vi "Start.vi"() -> ()   [LabVIEW 2016]
panel:
  in  "initial instruction string":string
  out "return count":u32=6435
  out "appended instruction string 2":string="dds reset\rdcp spi:CFR1=0x404000\rdcp spi:CFR2=0x80080\rdcp 0 spi:STP0=0x3FFF0000028F5C29\rdcp 1 spi:STP0=0x3FFF0000028F5C29\rdcp 0 spi:DRL=0x147C0118147BC1DB\rdcp 0 spi:DRSS=0xFFFFFFFF00000003\rdcp 0 spi:DRR=0x2D3E\rdcp 0 update:u-d\rdcp 0 update:+d\rdcp 1 spi:DRL=0x147AE148147AE148\rdcp 1 spi:DRSS=0xFFFFFFFF00000000\rdcp 1 spi:DRR=0xFFFF\rdcp 1 update:u-d\rdcp 1 update:+d\rdcp wait:1h:\rdcp wait::DROVER\rdcp 0 spi:DRL=0x147C51F1147C0118\rdcp 0 spi:DRSS=0xFFFFFFFF00000004\rdcp 0 spi:DRR=0x2F2F\rdcp 0 update:u-d\rdcp 0 update:+d\rdcp wait:1h:\rdcp wait::DROVER\rdcp 0 spi:DRL=0x147CB92D147C51F1\rdcp 0 spi:DRSS=0xFFFFFFFF00000017\rdcp 0 spi:DRR=0xD478\rdcp 0 update:u-d\rdcp 0 update:+d\rdcp wait:1h:\rdcp wait::DROVER\rdcp 0 spi:DRL=0x147D3CCC147CB92D\rdcp 0 spi:DRSS=0xFFFFFFFF00000009\rdcp 0 spi:DRR=0x4136\rdcp 0 update:u-d\rdcp 0 update:+d\rdcp wait:1h:\rdcp wait::DROVER\rdcp 0 spi:DRL=0x147DE446147D3CCC\rdcp 0 spi:DRSS=0xFFFFFFFF0000000D\rdcp 0 spi:DRR=0x4A07\rdcp 0 update:u-d\rdcp 0 update:+d\rdcp wait:1h:\rdcp wait::DROVER\rdcp 0 spi:DRL=0x147EB8D6147DE446\rdcp 0 spi:DRSS=0xFFFFFFFF0000002B\rdcp 0 spi:DRR=0xC0EC\rdcp 0 update:u-d\rdcp 0 update:+d\rdcp wait:1h:\rdcp wait::DROVER\rdcp 0 spi:DRL=0x147FC5C3147EB8D6\rdcp 0 spi:DRSS=0xFFFFFFFF00000006\rdcp 0 spi:DRR=0x1547\rdcp 0 update:u-d\rdcp 0 update:+d\rdcp wait:1h:\rdcp wait::DROVER\rdcp 0 spi:DRL=0x148118A1147FC5C3\rdcp 0 spi:DRSS=0xFFFFFFFF0000001C\rdcp 0 spi:DRR=0x4ECD\rdcp 0 update:u-d\rdcp 0 update:+d\rdcp wait:1h:\rdcp wait::DROVER\rdcp 0 spi:DRL=0x1482C174148118A1\rdcp 0 spi:DRSS=0xFFFFFFFF00000049\rdcp 0 spi:DRR=0xA3E0\rdcp 0 update:u-d\rdcp 0 update:+d\rdcp wait:1h:\rdcp wait::DROVER\rdcp 0 spi:DRL=0x1484D2A81482C174\rdcp 0 spi:DRSS=0xFFFFFFFF00000003\rdcp 0 spi:DRR=0x568\rdcp 0 update:u-d\rdcp 0 update:+d\rdcp wait:1h:\rdcp wait::DROVER\rdcp 0 spi:DRL=0x148760AD1484D2A8\rdcp 0 spi:DRSS=0xFFFFFFFF0000008C\rdcp 0 spi:DRR=0xCC25\rdcp 0 update:u-d\rdcp 0 update:+d\rdcp wait:1h:\rdcp wait::DROVER\rdcp 0 spi:DRL=0x148A8111148760AD\rdcp 0 spi:DRSS=0xFFFFFFFF00000049\rdcp 0 spi:DRR=0x56FB\rdcp 0 update:u-d\rdcp 0 update:+d\rdcp wait:1h:\rdcp wait::DROVER\rdcp 0 spi:DRL=0x148E48EB148A8111\rdcp 0 spi:DRSS=0xFFFFFFFF00000004\rdcp 0 spi:DRR=0x3F1\rdcp 0 update:u-d\rdcp 0 update:+d\rdcp wait:1h:\rdcp wait::DROVER\rdcp 0 spi:DRL=0x1492CA77148E48EB\rdcp 0 spi:DRSS=0xFFFFFFFF000000A0\rdcp 0 spi:DRR=0x8447\rdcp 0 update:u-d\rdcp 0 update:+d\rdcp wait:1h:\rdcp wait::DROVER\rdcp 0 spi:DRL=0x149811DB1492CA77\rdcp 0 spi:DRSS=0xFFFFFFFF000000D0\rdcp 0 spi:DRR=0x92C9\rdcp 0 update:u-d\rdcp 0 update:+d\rdcp wait:1h:\rdcp wait::DROVER\rdcp 0 spi:DRL=0x149E2175149811DB\rdcp 0 spi:DRSS=0xFFFFFFFF00000100\rdcp 0 spi:DRR=0x9D59\rdcp 0 update:u-d\rdcp 0 update:+d\rdcp wait:1h:\rdcp wait::DROVER\rdcp 0 spi:DRL=0x14A4EE42149E2175\rdcp 0 spi:DRSS=0xFFFFFFFF000000C7\rdcp 0 spi:DRR=0x6D05\rdcp 0 update:u-d\rdcp 0 update:+d\rdcp wait:1h:\rdcp wait::DROVER\rdcp 0 spi:DRL=0x14AC5D7114A4EE42\rdcp 0 spi:DRSS=0xFFFFFFFF00000019\rdcp 0 spi:DRR=0xC87\rdcp 0 update:u-d\rdcp 0 update:+d\rdcp wait:1h:\rdcp wait::DROVER\rdcp 0 spi:DRL=0x14B4443314AC5D71\rdcp 0 spi:DRSS=0xFFFFFFFF00000021\rdcp 0 spi:DRR=0xF8F\rdcp 0 update:u-d\rdcp 0 update:+d\rdcp wait:1h:\rdcp wait::DROVER\rdcp 0 spi:DRL=0x14BC6A7F14B44433\rdcp 0 spi:DRSS=0xFFFFFFFF0000014D\rdcp 0 spi:DRR=0x9838\rdcp 0 update:u-d\rdcp 0 update:+d\rdcp wait:1h:\rdcp wait::DROVER\rdcp 0 spi:DRL=0x14C490CB14BC6A7F\rdcp 0 spi:DRSS=0xFFFFFFFF0000014D\rdcp 0 spi:DRR=0x9838\rdcp 0 update:u-d\rdcp 0 update:+d\rdcp wait:1h:\rdcp wait::DROVER\rdcp 0 spi:DRL=0x14CC778D14C490CB\rdcp 0 spi:DRSS=0xFFFFFFFF00000021\rdcp 0 spi:DRR=0xF8F\rdcp 0 update:u-d\rdcp 0 update:+d\rdcp wait:1h:\rdcp wait::DROVER\rdcp 0 spi:DRL=0x14D3E6BC14CC778D\rdcp 0 spi:DRSS=0xFFFFFFFF00000019\rdcp 0 spi:DRR=0xC87\rdcp 0 update:u-d\rdcp 0 update:+d\rdcp wait:1h:\rdcp wait::DROVER\rdcp 0 spi:DRL=0x14DAB38914D3E6BC\rdcp 0 spi:DRSS=0xFFFFFFFF000000C7\rdcp 0 spi:DRR=0x6D05\rdcp 0 update:u-d\rdcp 0 update:+d\rdcp wait:1h:\rdcp wait::DROVER\rdcp 0 spi:DRL=0x14E0C32314DAB389\rdcp 0 spi:DRSS=0xFFFFFFFF00000100\rdcp 0 spi:DRR=0x9D59\rdcp 0 update:u-d\rdcp 0 update:+d\rdcp wait:1h:\rdcp wait::DROVER\rdcp 0 spi:DRL=0x14E60A8714E0C323\rdcp 0 spi:DRSS=0xFFFFFFFF000000D0\rdcp 0 spi:DRR=0x92C9\rdcp 0 update:u-d\rdcp 0 update:+d\rdcp wait:1h:\rdcp wait::DROVER\rdcp 0 spi:DRL=0x14EA8C1314E60A87\rdcp 0 spi:DRSS=0xFFFFFFFF000000A0\rdcp 0 spi:DRR=0x8447\rdcp 0 update:u-d\rdcp 0 update:+d\rdcp wait:1h:\rdcp wait::DROVER\rdcp 0 spi:DRL=0x14EE53ED14EA8C13\rdcp 0 spi:DRSS=0xFFFFFFFF00000004\rdcp 0 spi:DRR=0x3F1\rdcp 0 update:u-d\rdcp 0 update:+d\rdcp wait:1h:\rdcp wait::DROVER\rdcp 0 spi:DRL=0x14F1745114EE53ED\rdcp 0 spi:DRSS=0xFFFFFFFF00000049\rdcp 0 spi:DRR=0x56FB\rdcp 0 update:u-d\rdcp 0 update:+d\rdcp wait:1h:\rdcp wait::DROVER\rdcp 0 spi:DRL=0x14F4025514F17451\rdcp 0 spi:DRSS=0xFFFFFFFF0000008C\rdcp 0 spi:DRR=0xCC25\rdcp 0 update:u-d\rdcp 0 update:+d\rdcp wait:1h:\rdcp wait::DROVER\rdcp 0 spi:DRL=0x14F6138A14F40255\rdcp 0 spi:DRSS=0xFFFFFFFF00000003\rdcp 0 spi:DRR=0x568\rdcp 0 update:u-d\rdcp 0 update:+d\rdcp wait:1h:\rdcp wait::DROVER\rdcp 0 spi:DRL=0x14F7BC5D14F6138A\rdcp 0 spi:DRSS=0xFFFFFFFF00000049\rdcp 0 spi:DRR=0xA3E0\rdcp 0 update:u-d\rdcp 0 update:+d\rdcp wait:1h:\rdcp wait::DROVER\rdcp 0 spi:DRL=0x14F90F3B14F7BC5D\rdcp 0 spi:DRSS=0xFFFFFFFF0000001C\rdcp 0 spi:DRR=0x4ECD\rdcp 0 update:u-d\rdcp 0 update:+d\rdcp wait:1h:\rdcp wait::DROVER\rdcp 0 spi:DRL=0x14FA1C2814F90F3B\rdcp 0 spi:DRSS=0xFFFFFFFF00000006\rdcp 0 spi:DRR=0x1547\rdcp 0 update:u-d\rdcp 0 update:+d\rdcp wait:1h:\rdcp wait::DROVER\rdcp 0 spi:DRL=0x14FAF0B814FA1C28\rdcp 0 spi:DRSS=0xFFFFFFFF0000002B\rdcp 0 spi:DRR=0xC0EC\rdcp 0 update:u-d\rdcp 0 update:+d\rdcp wait:1h:\rdcp wait::DROVER\rdcp 0 spi:DRL=0x14FB983214FAF0B8\rdcp 0 spi:DRSS=0xFFFFFFFF0000000D\rdcp 0 spi:DRR=0x4A07\rdcp 0 update:u-d\rdcp 0 update:+d\rdcp wait:1h:\rdcp wait::DROVER\rdcp 0 spi:DRL=0x14FC1BD114FB9832\rdcp 0 spi:DRSS=0xFFFFFFFF00000009\rdcp 0 spi:DRR=0x4136\rdcp 0 update:u-d\rdcp 0 update:+d\rdcp wait:1h:\rdcp wait::DROVER\rdcp 0 spi:DRL=0x14FC830D14FC1BD1\rdcp 0 spi:DRSS=0xFFFFFFFF00000017\rdcp 0 spi:DRR=0xD478\rdcp 0 update:u-d\rdcp 0 update:+d\rdcp wait:1h:\rdcp wait::DROVER\rdcp 0 spi:DRL=0x14FCD3E614FC830D\rdcp 0 spi:DRSS=0xFFFFFFFF00000004\rdcp 0 spi:DRR=0x2F2F\rdcp 0 update:u-d\rdcp 0 update:+d\rdcp wait:1h:\rdcp wait::DROVER\rdcp 0 spi:DRL=0x14FD132314FCD3E6\rdcp 0 spi:DRSS=0xFFFFFFFF00000003\rdcp 0 spi:DRR=0x2D3E\rdcp 0 update:u-d\rdcp 0 update:+d\rdcp wait:1h:\rdcp wait::DROVER\rdcp 0 spi:DRL=0x14FD448E14FD1323\rdcp 0 spi:DRSS=0xFFFFFFFF00000002\rdcp 0 spi:DRR=0x2699\rdcp 0 update:u-d\rdcp 0 update:+d\rdcp wait:1h:\rdcp wait::DROVER\rdcp start\r"
  out "error out":errorcluster={"status"=TRUE, "code"=-1073807339, "source"="VISA Read in FlexDDS-NG_USB_Example.vi"}
  out "read buffer":string
  in  "FlexDDS-NG USB VISA resource name (COM)":refnum<visa-resource-name>="COM5"
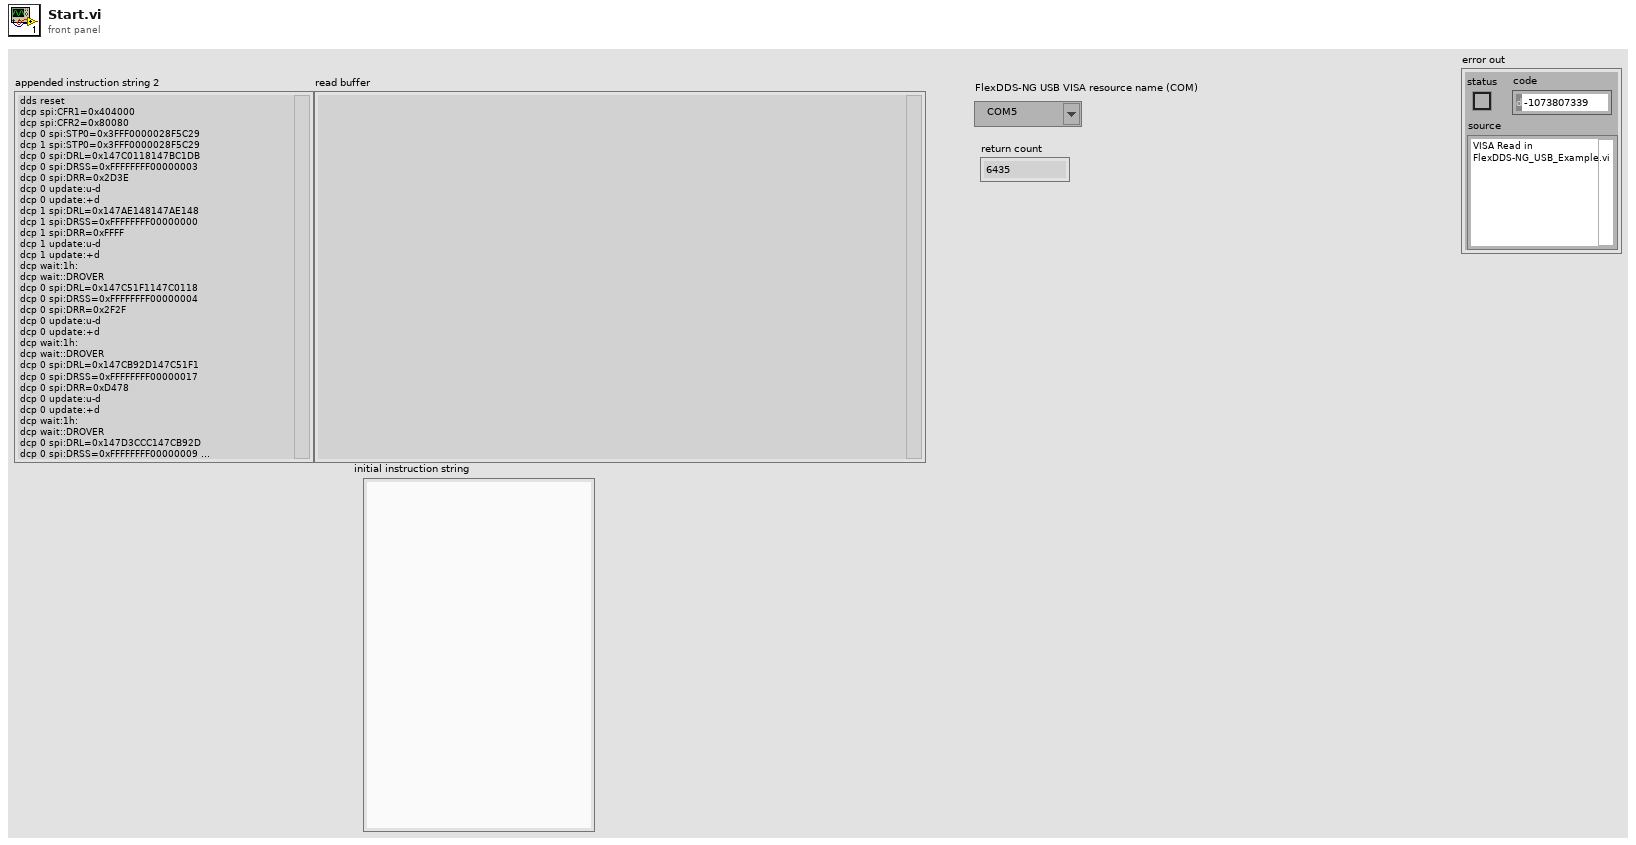
[diagram p1: front panel]
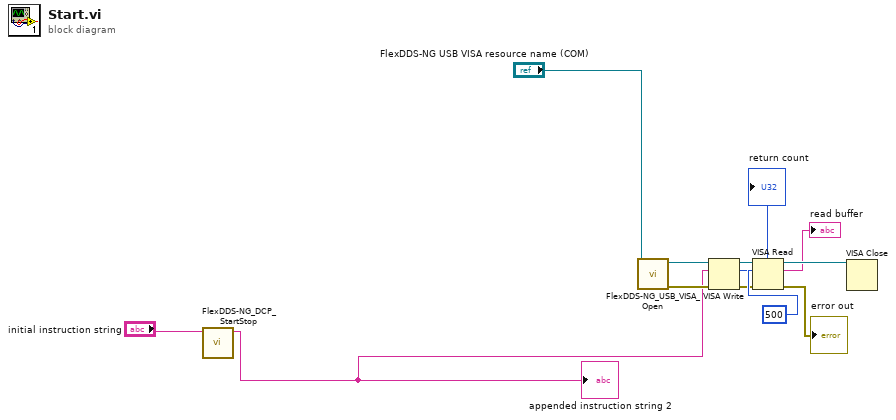
[diagram p0: block diagram]
diagram:
  n1 = call "FlexDDS-NG_DCP_StartStop.vi"("initial instruction string"="initial instruction string") -> ("appended instruction string"=w2:string)  [unwired: 10 in]
  "appended instruction string 2" <- w2
  n2 = call "FlexDDS-NG_USB_VISA_Open.vi"("FlexDDS-NG USB VISA resource name (COM)"="FlexDDS-NG USB VISA resource name (COM)") -> ("error out"=w6:errorcluster, "FlexDDS-NG USB VISA resource name out"=w8:refnum<visa-resource-name>)  [unwired: 9 in]
  n3 = VISA Write(VISA resource name=w8, write buffer=w2, error in (no error)=w6) -> (VISA resource name out=w9:refnum<visa-resource-name>, return count=→"return count":u32, error out=w5:errorcluster)
  n4 = VISA Read(VISA resource name=w9, byte count=u32 500, error in (no error)=w5) -> (VISA resource name out=w12:refnum<visa-resource-name>, read buffer=→"read buffer":string, error out=→"error out":errorcluster)  [unwired: 1 out]
  n5 = VISA Close(VISA resource name=w12) -> ()  [unwired: 1 in, 1 out]
